vi "Step Add IR W Parameters.vi"(0 "VISA resource name":refnum<visa-resource-name>, 1 "IR Test Parameters in":T1={"Voltage (1000)"=1000, "High Limit(0.0, 0.5 - 50000 Megohms) (5)"=0.0, "Low Limit(0.1 - 50000 Megohms) (0)"=0.1, "Ramp Up Time (0.1 - 999.9 seconds) (0.1)"=0.1, "Delay Time (0.0, 1.0 - 999.9 seconds) (0.5)"=0.5, "Ramp Down Time (0.0 - 999.9 seconds) (0) "=0.0, "Charge LO (0)"=0.0, "Auto Charge LO (F: Off)"=FALSE, "Dwell Time (0.0, 1.0 - 999.9 seconds) (0.5)"=0.5} {"Dwell Time (0.0, 1.0 - 999.9 seconds) (0.5)" format="%.1f"; "Ramp Down Time (0.0 - 999.9 seconds) (0)" format="%.1f"; "Charge LO (0)" format="%.2f"; "Delay Time (0.0, 1.0 - 999.9 seconds) (0.5)" format="%.1f"; "Ramp Up Time (0.1 - 999.9 seconds) (0.1)" format="%.1f"; "Low Limit(0.1 - 50000 Megohms) (0)" format="%.1f"; "High Limit(0.0, 0.5 - 50000 Megohms) (5)" format="%.1f"}, 2 "Internal Scanner Exists?":bool, 3 "Scanner Settings":T2={"Scan1"=1, "Scan2"=1, "Scan3"=1, "Scan4"=1, "Scan5"=1, "Scan6"=1, "Scan7"=1, "Scan8"=1, "Scan9"=1, "Scan10"=1, "Scan11"=1, "Scan12"=1, "Scan13"=1, "Scan14"=1, "Scan15"=1, "Scan16"=1} {"Scan16" scale=0.0..2.0; "Scan15" scale=0.0..2.0; "Scan14" scale=0.0..2.0; "Scan13" scale=0.0..2.0; "Scan12" scale=0.0..2.0; "Scan11" scale=0.0..2.0; "Scan10" scale=0.0..2.0; "Scan9" scale=0.0..2.0; "Scan8" scale=0.0..2.0; "Scan7" scale=0.0..2.0; "Scan6" scale=0.0..2.0; "Scan5" scale=0.0..2.0; "Scan4" scale=0.0..2.0; "Scan3" min=0 max=2 scale=0.0..2.0; "Scan2" min=0 max=2 scale=0.0..2.0; "Scan1" min=0 max=2 scale=0.0..2.0}, 7 "Step Selection (1-200)":i32=1, 9 "Add Step":bool, 11 "error in (no error)":errorcluster) -> (4 "VISA resource name out":refnum<visa-resource-name>, 15 "error out":errorcluster)   [LabVIEW 2020, in "Associated Research 78XX Series.lvlib"]
doc: "Set the desired memory location to IR mode with the specified parameters."
uses:
  <instrlib>/Associated Research 78XX Series/Associated Research 78XX Series.lvlib
  <instrlib>/Associated Research 78XX Series/Public/Configure/Steps/Low Level/Scanner Settings.ctl
  <instrlib>/Associated Research 78XX Series/Public/Configure/Steps/Low Level/IR Test Parameters.ctl
panel:
  # "Add"
  # "Edit"
  # "On\nOff"
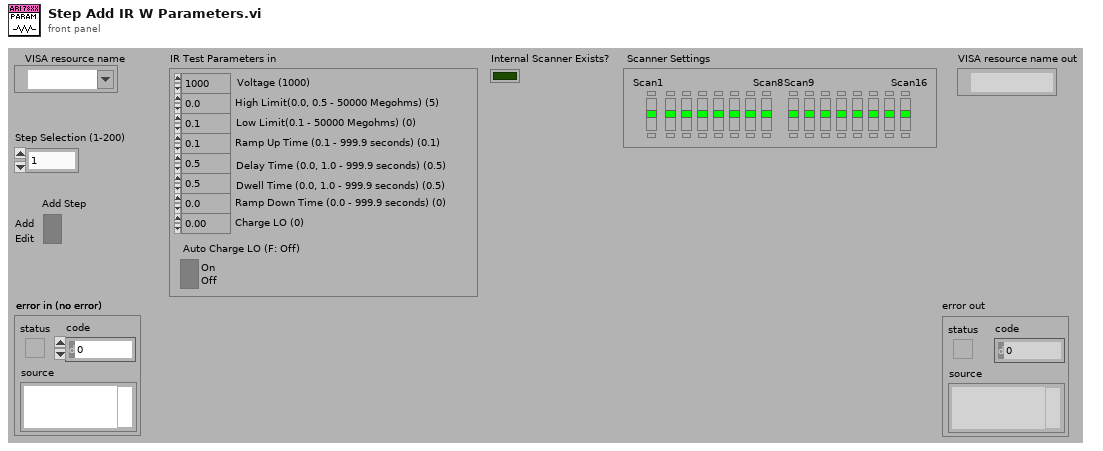
[diagram p1: front panel]
types:
  T1 = typedef "Associated Research 78XX Series.lvlib/IR Test Parameters.ctl" = cluster{"Voltage (1000)":i32, "High Limit(0.0, 0.5 - 50000 Megohms) (5)":dbl, "Low Limit(0.1 - 50000 Megohms) (0)":dbl, "Ramp Up Time (0.1 - 999.9 seconds) (0.1)":dbl, "Delay Time (0.0, 1.0 - 999.9 seconds) (0.5)":dbl, "Ramp Down Time (0.0 - 999.9 seconds) (0) ":dbl, "Charge LO (0)":dbl, "Auto Charge LO (F: Off)":bool, "Dwell Time (0.0, 1.0 - 999.9 seconds) (0.5)":dbl}
  T2 = typedef "Associated Research 78XX Series.lvlib/Scanner Settings.ctl" = cluster{"Scan1":i32, "Scan2":i32, "Scan3":i32, "Scan4":i32, "Scan5":i32, "Scan6":i32, "Scan7":i32, "Scan8":i32, "Scan9":i32, "Scan10":i32, "Scan11":i32, "Scan12":i32, "Scan13":i32, "Scan14":i32, "Scan15":i32, "Scan16":i32}
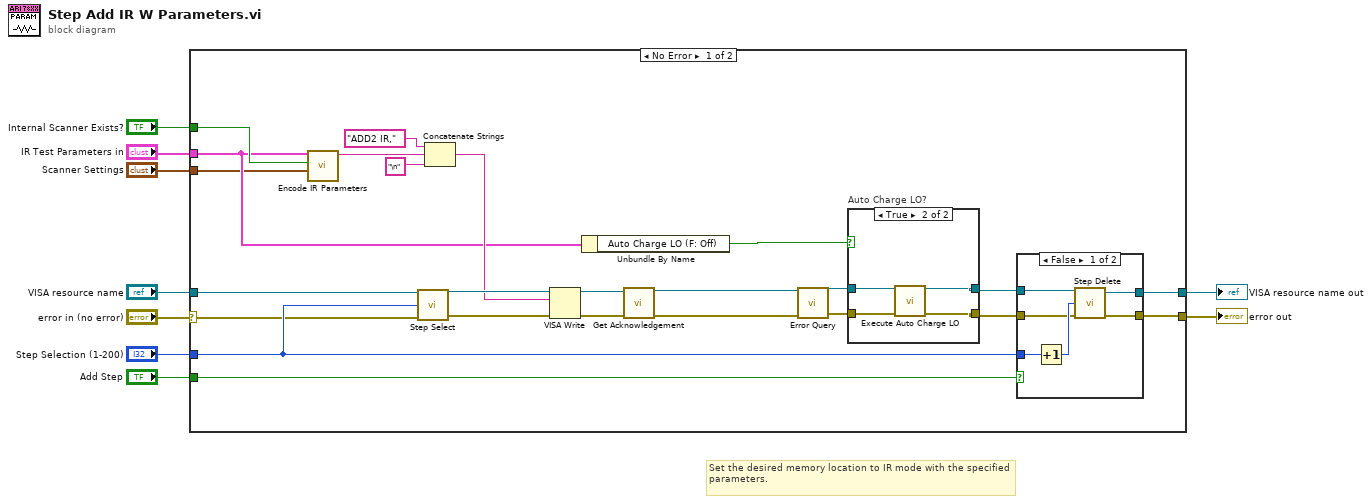
[diagram p0: block diagram]
diagram:
  # "Set the desired memory location to IR mode with the specified parameters."
  n1 = case shown="No Error" "error in (no error)" {
    selector: "error in (no error)" -> [w15 w49]
    tunnel: [w30 w49] -> w8
    tunnel: [w29 w48] -> w6
    tunnel: "VISA resource name" -> [w16 w48]
    tunnel: "Step Selection (1-200)" -> [w31 _]
    tunnel: "Add Step" -> [w28 _]
    tunnel: "IR Test Parameters in" -> [w11 _]
    tunnel: "Internal Scanner Exists?" -> [w27 _]
    tunnel: "Scanner Settings" -> [w10 _]
    frame No Error {
      n2 = call <instrlib>:"Encode IR Parameters.vi"("Scanner Settings in"=w10, "Internal Scanner Exists?"=w27, "IR Test Parameters in"=w11) -> ("ADD command"=w26:string)  [unwired: 6 in, 2 out]
      n3 = call <instrlib>:"Step Select.vi"("VISA resource name"=w16, "Step Number (1)"=w31, "error in (no error)"=w15) -> ("VISA resource name out"=w32:refnum<visa-resource-name>, "error out"=w33:errorcluster)  [unwired: 11 in]
      n4 = Concatenate Strings("ADD2 IR," ("string"), w26, "\n" ("string")) -> (w24:string)
      n5 = VISA Write(VISA resource name=w32, write buffer=w24, error in (no error)=w33) -> (VISA resource name out=w13:refnum<visa-resource-name>, error out=w12:errorcluster)  [unwired: 1 out]
      n6 = Unbundle By Name(w11) -> ("Auto Charge LO (F: Off)"=w19:bool)
      n7 = call <instrlib>:"Get Acknowledgement.vi"("VISA resource name"=w13, "error in (no error)"=w12) -> ("VISA resource name out"=w18:refnum<visa-resource-name>, "error out"=w17:errorcluster)  [unwired: 12 in]
      n8 = call <instrlib>:"Error Query.vi"("VISA resource name"=w18, "error in (no error)"=w17) -> ("VISA resource name out"=w23:refnum<visa-resource-name>, "error out"=w22:errorcluster)  [unwired: 10 in, 2 out]
      n9 = case "Auto Charge LO?" shown="True" w19 {
        tunnel: w23 -> [w35 w39]
        tunnel: w22 -> [w34 w38]
        tunnel: [w34 w36] -> w21
        tunnel: [w35 w37] -> w20
        frame False {
        }
        frame True {
          n10 = call <instrlib>:"Execute Auto Charge LO.vi"("VISA resource name"=w39, "error in (no error)"=w38) -> ("VISA resource name out"=w37:refnum<visa-resource-name>, "error out"=w36:errorcluster)  [unwired: 12 in]
        }
      }
      n11 = case shown="False" w28 {
        tunnel: w31 -> [w45 _]
        tunnel: w21 -> [w43 w46]
        tunnel: w20 -> [w42 w47]
        tunnel: [w41 w46] -> w30
        tunnel: [w40 w47] -> w29
        frame False {
          n12 = Increment(x=w45) -> (x+1=w44:i32)
          n13 = call <instrlib>:"Step Delete.vi"("VISA resource name"=w42, "Step Number (0 = Active Step)"=w44, "error in (no error)"=w43) -> ("VISA resource name out"=w40:refnum<visa-resource-name>, "error out"=w41:errorcluster)  [unwired: 11 in]
        }
        frame True {
        }
      }
    }
    frame Error {
    }
  }
  "error out" <- w8
  "VISA resource name out" <- w6
